vi "FilesNameDefine_V0.vi"() -> (0 "date/time string":string, 1 "Result File Name":string)   [LabVIEW 2021]
doc: "This vi helps to convert time information to string and combine it with a predefined file name."
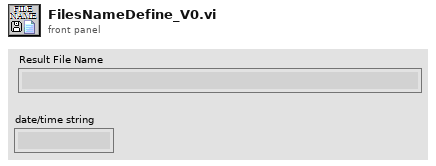
[diagram p1: front panel]
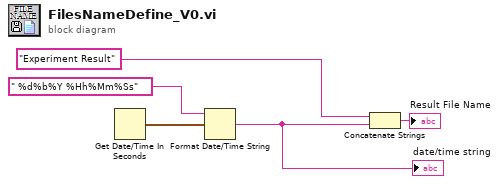
[diagram p0: block diagram]
diagram:
  n1 = Get Date/Time In Seconds() -> (seconds since 1Jan1904=w5:timestamp)
  n2 = Format Date/Time String(time format string (%c)=" %d%b%Y %Hh%Mm%Ss", seconds (now)=w5) -> (date/time string=w3:string)  [unwired: 1 in]
  "date/time string" <- w3
  n3 = Concatenate Strings("Experiment Result", w3) -> (→"Result File Name":string)
